vi "NetworkUDP_Send.vi"(7 "remote port":u16=5801, 8 "error in (no error)":errorcluster, 9 "timeout ms (25000)":i32=1000, 10 "IP4 Address":u32, 11 "data string":string) -> (0 "error out":errorcluster, 2 "UDP Network Connection out":refnum<k16>, 3 "Consec Err":i32)   [LabVIEW 2019, in "Trajectory_Library.lvlib"]
uses:
  Trajectory_Library.lvlib
panel:
  # "UDP WRITE"
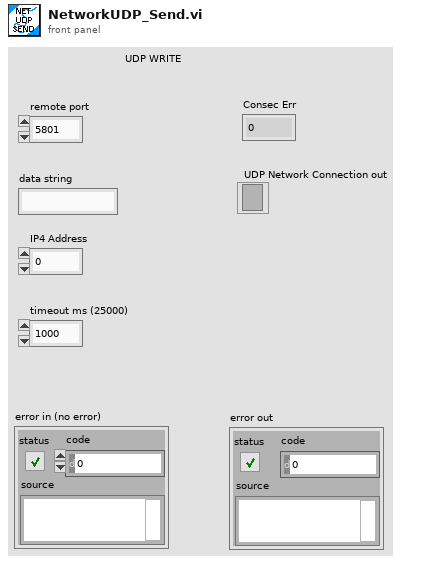
[diagram p1: front panel]
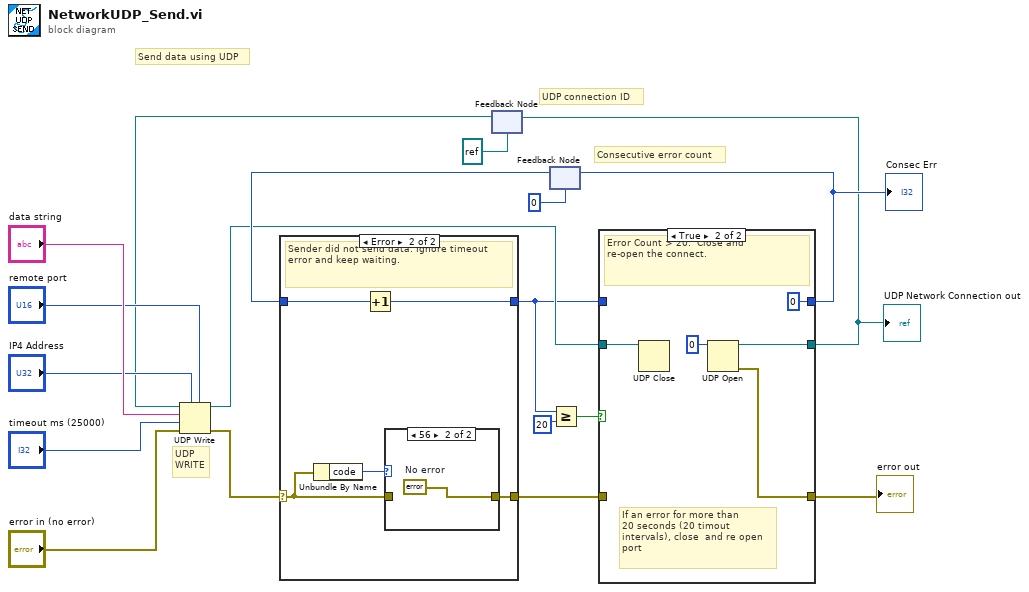
[diagram p0: block diagram]
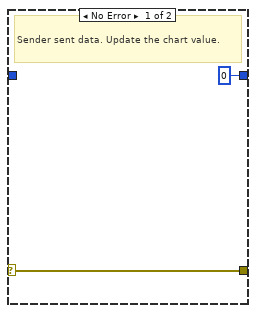
[diagram p3: hidden frame]
diagram:
  # "Send data using UDP"
  # "UDP connection ID"
  # "Consecutive error count"
  # "UDP\nWRITE"
  n1 = feedback #1(refnum<k16> refnum ("port")) -> (w4:refnum<k16>)
  n2 = UDP Write(address="IP4 Address", port or service name="remote port", connection ID=w4, data in="data string", 8:"error in (no error)", 9:"timeout ms (25000)") -> (error out=w6:errorcluster, 3:w5:refnum<k16>)
  n3 = feedback #2(0) -> (w8:i32)
  n4 = case shown="Error" w6 {
    selector: w6 -> [w20 w24]
    tunnel: [w20 w23] -> w13
    tunnel: w8 -> [_ w22]
    tunnel: [0 w21] -> w3
    frame No Error {
      (unwired) 0
      # "Sender sent data. Update the chart value."
    }
    frame Error {
      # "Sender did not send data. Ignore timeout error and keep waiting."
      n5 = Unbundle By Name(w24) -> ("code"=w25:i32)
      n6 = Increment(x=w22) -> (x+1=w21:i32)
      n7 = case shown="56" w25 {
        tunnel: w24 -> [w26 _]
        tunnel: [w26 w27] -> w23
        frame Default {
        }
        frame 56 {
          w27 = errorcluster {"status"=FALSE, "code"=0, "source"=""}  # No error
        }
      }
    }
  }
  n8 = Greater Or Equal?(x=w3, y=20) -> (x >= y?=w12:bool)
  n9 = case shown="True" w12 {
    tunnel: w3 -> [w30 _]
    tunnel: [w30 0] -> w10
    tunnel: w5 -> [w29 w35]
    tunnel: [w29 w34] -> w1
    tunnel: w13 -> [w28 _]
    tunnel: [w28 w33] -> w14
    frame False {
      # "Not greater than\n200 consecutive\nerrors"
      # "Not greater than 20 consecutive errrors.  Don't do anyting yet."
    }
    frame True {
      # "If an error for more than\n20 seconds (20 timout\nintervals), close  and re open \nport"
      # "Error Count > 20.  Close and \nre-open the connect."
      n10 = UDP Close(connection ID=w35) -> ()  [unwired: 1 in, 2 out]
      n11 = UDP Open(11:u16 0 ("port")) -> (port=w34:refnum<k16>, 0:w33:errorcluster)  [unwired: 4 in, 1 out]
    }
  }
  "UDP Network Connection out" <- w1
  "Consec Err" <- w10
  "error out" <- w14
  n12 = feedback-in #1(w1) -> ()
  n13 = feedback-in #2(w10) -> ()
